vi "Abort.vi"(8 "error in (no error)":errorcluster, 11 "LUnit Test Suite in":refnum<class "LUnit Test Suite.lvclass">) -> (0 "error out":errorcluster)   [LabVIEW 2020, in "LUnit Test Suite.lvclass"]
uses:
  LUnit Test Suite.lvclass
  LUnit Test Suite.lvclass/LUnit Test Suite.ctl
  Core/Runnable/Runnable.lvclass
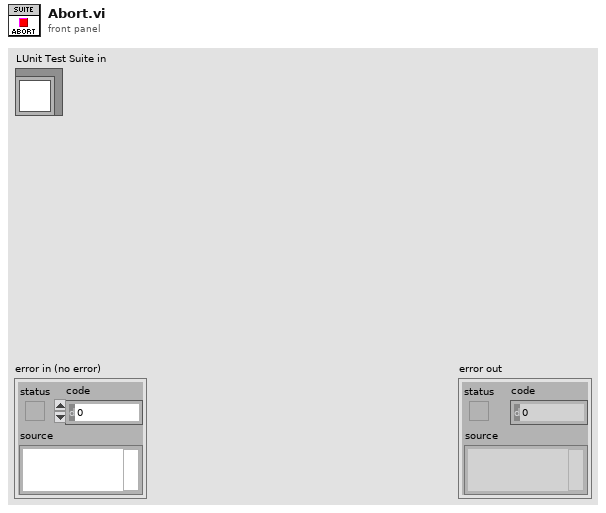
[diagram p1: front panel]
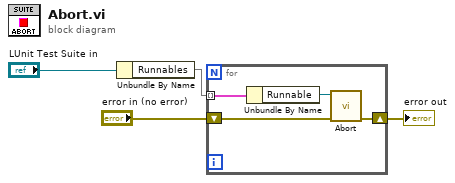
[diagram p0: block diagram]
diagram:
  n1 = Unbundle By Name("LUnit Test Suite in") -> ("Runnables"=w3:map{string, refnum<class "Runnable.lvclass">})
  n2 = for {
    tunnel: w3 -> [w8] mode=indexing
    shift-right: [w5] -> w1
    shift-left: "error in (no error)" -> [w6]
    n3 = Unbundle By Name(w8) -> ("Runnable"=w7:refnum<class "Runnable.lvclass">)
    n4 = call-dynamic "Abort.vi"("error in (no error)"=w6, "Runnable in"=w7) -> ("error out"=w5:errorcluster)  [unwired: 9 in]
  }
  "error out" <- w1
